vi "DrawTriangle3D.vi"(9 "Display":T1={"Mode"=enum."Inherit Value", "PointSize"=1.0, "LineWidth"=1.0}, 10 "Color":T4={"Alpha"=1.0, "Color"=16448250} {"Alpha" min=0.0 max=1.0 scale=0.0..1.0}, 11 "Triangles":T2[](array[typedef])) -> ()   [LabVIEW 2014]
uses:
  TypeDefs/Color.ctl
  TypeDefs/TriangleFace.ctl
  TypeDefs/Point3D.ctl
  <vilib>/picture/3D Picture Control/Object/Create Object (name).vi
  <vilib>/picture/3D Picture Control/Object/Add Object (no reference).vi
  <vilib>/picture/3D Picture Control/NI_3D Picture Control.lvlib
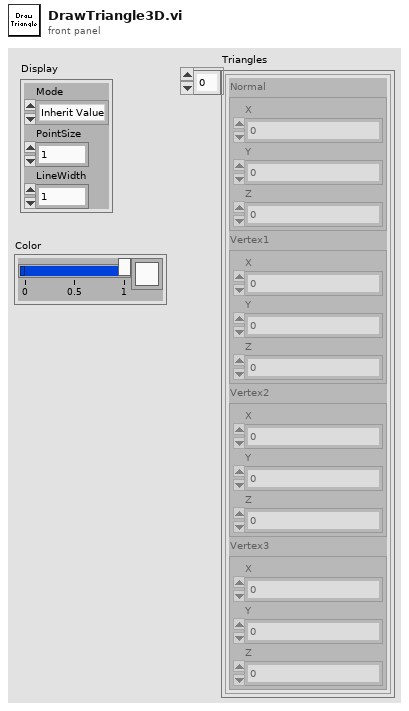
[diagram p1: front panel]
types:
  T1 = cluster{"Mode":enum16{"Inherit Value", "Points", "Wireframe", "Polygons"}, "PointSize":sgl, "LineWidth":sgl}
  T2 = typedef "TriangleFace.ctl" = cluster{"Normal":T3, "Vertex1":T3, "Vertex2":T3, "Vertex3":T3}
  T3 = typedef "Point3D.ctl" = cluster{"X":sgl, "Y":sgl, "Z":sgl}
  T4 = typedef "Color.ctl" = cluster{"Alpha":dbl, "Color":u32}
  T5 = enum16{"New", "Find", "FindPattern", "GetTable", "Clear"}
  T6 = enum16{"Inherit Value", "Points", "Wireframe", "Polygons"}
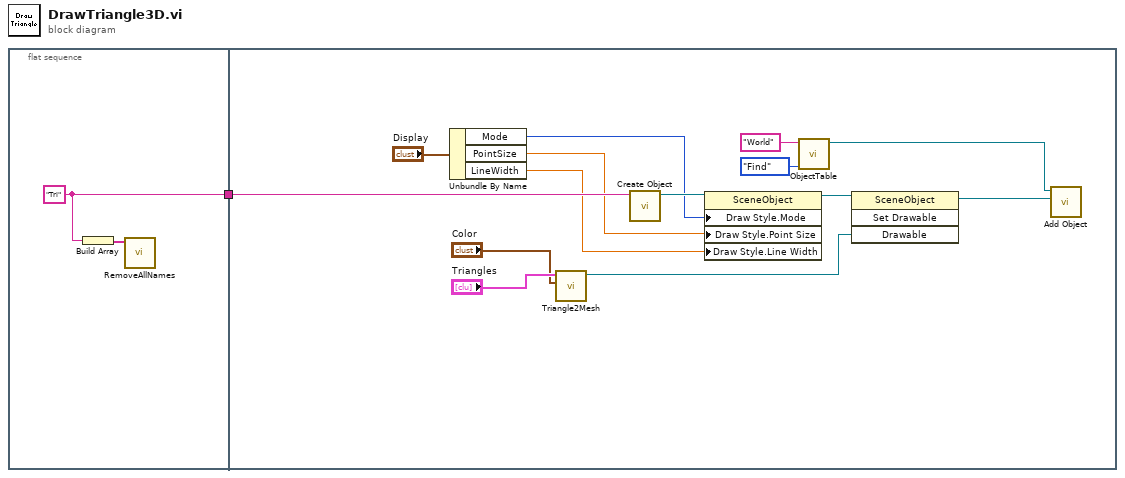
[diagram p0: block diagram]
diagram:
  n1 = flat-sequence {
    tunnel: [w2] -> w1
    tunnel: w1 -> [w8]
    frame #0 {
      w2 = "Tri" ("string")
      n2 = Build Array(w2) -> (w3:string[])
      n3 = call "RemoveAllNames.vi"("Names"=w3) -> ()  [unwired: 11 in]
    }
    frame #1 {
      n4 = Unbundle By Name("Display") -> ("Mode"=w6:T6, "PointSize"=w5:sgl, "LineWidth"=w4:sgl)
      n5 = call "Triangle2Mesh.vi"("Color"="Color", "Triangles"="Triangles") -> ("Refnum"=w9:refnum<vi>)  [unwired: 9 in]
      n6 = call-poly <vilib>:"Create Object.vi"("Name"=w8) -> ("Scene:New Object"=w12:refnum<vi>)  [unwired: 9 in, 1 out]
      n7 = property class="SceneObject"(reference=w12, "Draw Style.Mode"=w6, "Draw Style.Point Size"=w5, "Draw Style.Line Width"=w4) -> (reference out=w13:refnum<vi>)  [unwired: 1 in, 1 out]
      n8 = call "ObjectTable.vi"("ObjectStoreSelector"=T5."Find", "Name"="World") -> ("ObjectRef"=w14:refnum<vi>)  [unwired: 5 in, 4 out]
      n9 = invoke class="SceneObject" method="Set Drawable"(reference=w13, "Drawable"=w9) -> (reference out=w15:refnum<vi>)  [unwired: 2 in, 3 out]
      n10 = call-poly <vilib>:"Add Object.vi"("New Object In"=w15, "Scene Object In"=w14) -> ()  [unwired: 8 in, 2 out]
    }
  }
